vi "DBL Array To Multi-Item Text.vi"(10 "DBL Array":dbl[](array[numeric])) -> (2 "Multi-Item Text":cluster{string[]}[](array[cluster]))   [LabVIEW 2024]
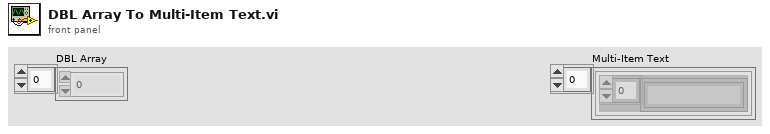
[diagram p1: front panel]
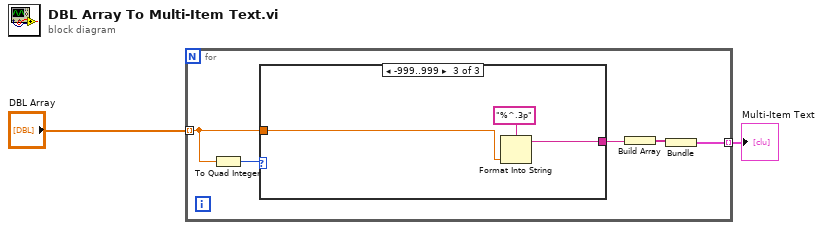
[diagram p0: block diagram]
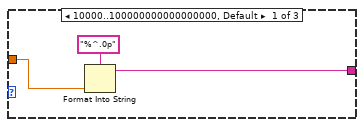
[diagram p2: hidden frame]
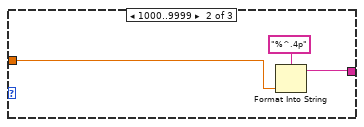
[diagram p3: hidden frame]
diagram:
  n1 = for {
    tunnel: "DBL Array" -> [w7] mode=indexing
    tunnel: [w3] -> w1 mode=indexing
    n2 = To Quad Integer(1:w7) -> (0:w6:i64)
    n3 = case shown="-999..999" w6 {
      tunnel: [w8 w12 w15] -> w5
      tunnel: w7 -> [w9 w11 w14]
      frame 10000..100000000000000000, Default {
        n4 = Format Into String(format string="%^.0p", w9) -> (resulting string=w8:string)  [unwired: 2 in, 1 out]
      }
      frame 1000..9999 {
        n5 = Format Into String(format string="%^.4p", w11) -> (resulting string=w12:string)  [unwired: 2 in, 1 out]
      }
      frame -999..999 {
        n6 = Format Into String(format string="%^.3p", w14) -> (resulting string=w15:string)  [unwired: 2 in, 1 out]
      }
    }
    n7 = Build Array(w5) -> (w4:string[])
    n8 = Bundle(w4) -> (w3:cluster{string[]})  [unwired: 1 in]
  }
  "Multi-Item Text" <- w1
